vi "number to decimal_0.vi"() -> ()   [LabVIEW 2015]
panel:
  in  "Tab Control":enum32{"Page 1", "Page 2"}(tab)
  in  "number":u32
  out "Binarry  value":bool[](array[boolean])
  in  "stop":bool
  # "Covert number to Binary value"
  # "Pardeep Kumar"
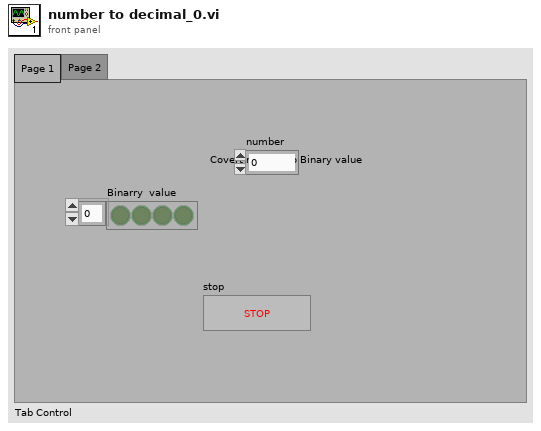
[diagram p1: front panel]
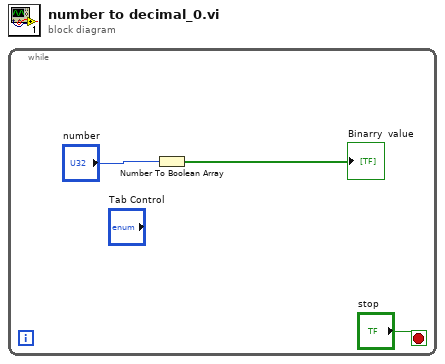
[diagram p0: block diagram]
diagram:
  n1 = while {
    stop <- "stop" stop-if-true
    n2 = Number To Boolean Array(number="number") -> (Boolean array=→"Binarry  value":bool[])
  }
